vi "testserverstream.vi"() -> ()   [LabVIEW 2016]
uses:
  dllwrapper/tls data user event.ctl
  dllwrapper/tls new socket user event.ctl
  dllwrapper/tls action complete user event.ctl
  dllwrapper/async tls.lvlib
  lvasynctls.dll
panel:
  out "buffer":string
  out "streamreaderr":i32
  out "read size?":u64
  out "error string":string
  out "length":u32
  out "errstring":string
  out "anyconn 2":u32 format="%.0x"
  out "anyconn":u64 format="%.0x"
  out "options":errorcluster
  out "data":string
  out "bad connection":u64
  out "request type 3":u8 format="%.0x"
  out "request ID 3":u32 format="%.0x"
  out "error code 3":i32 format="%.0x"
  out "request type 2":u8 format="%.0x"
  out "request ID 2":u32 format="%.0x"
  out "error code 2":i32 format="%.0x"
  out "error code":i32
  out "request ID":u32 format="%.0x"
  out "request type":u32 format="%.0x"
  out "error out 10":errorcluster
  out "error out 9":errorcluster
  out "error out 6":errorcluster
  out "error out 5":errorcluster
  out "error out 4":errorcluster
  out "error out 3":errorcluster
  out "error out 2":errorcluster
  # "read result"
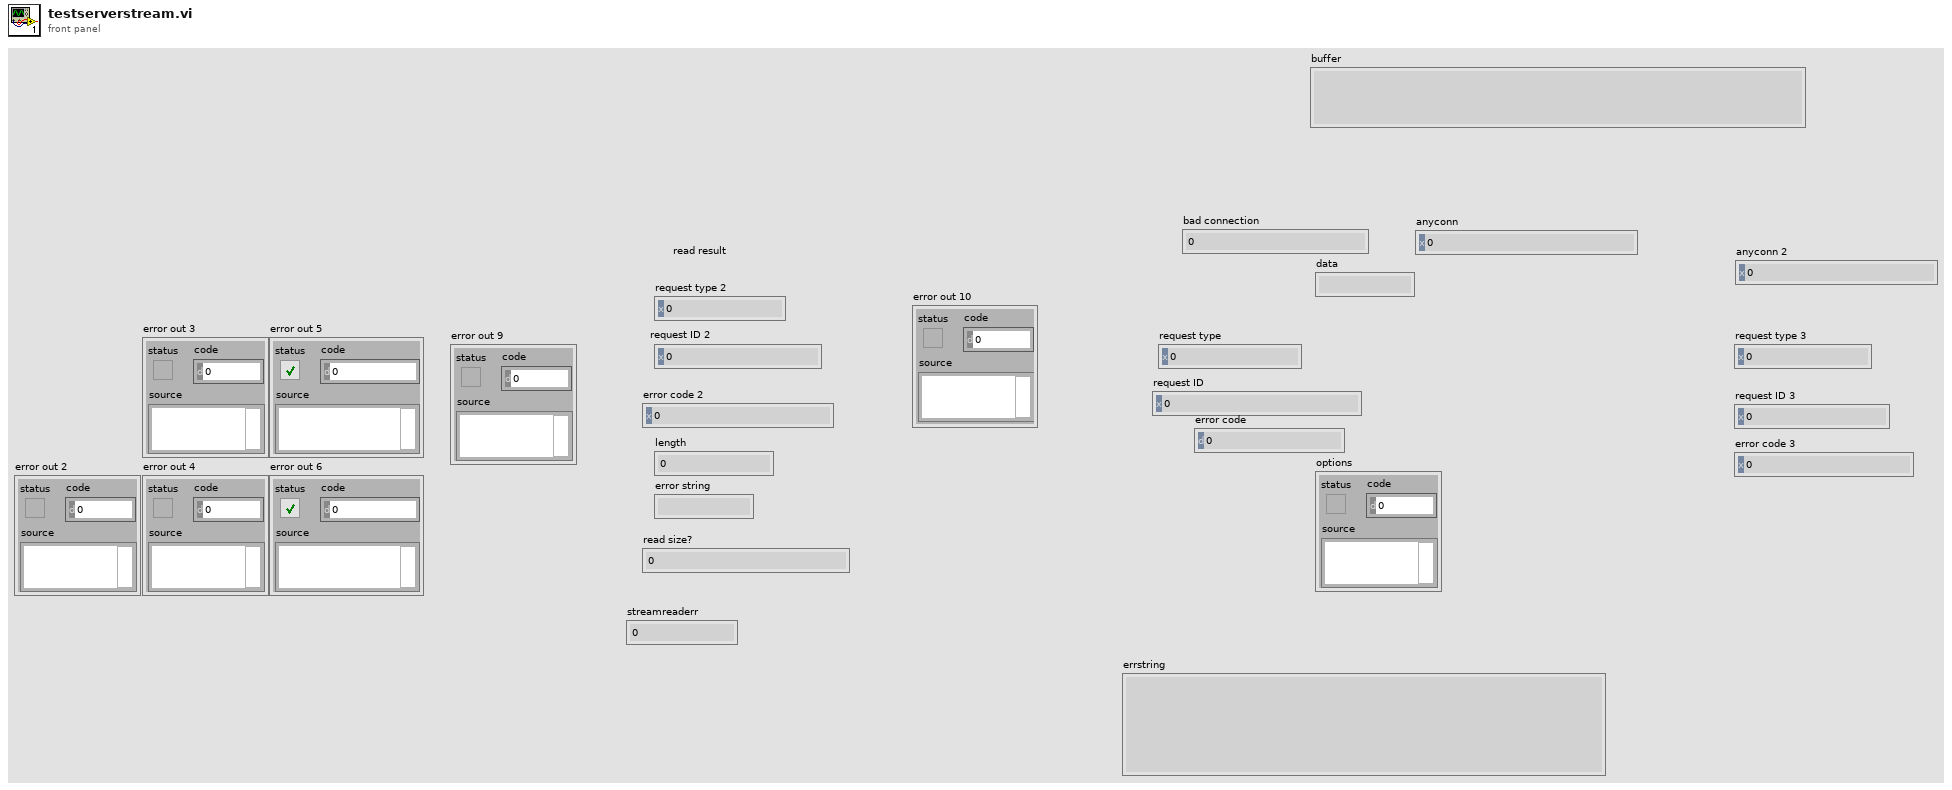
[diagram p1: front panel]
types:
  T1 = typedef "async tls.lvlib/tls action complete user event.ctl" = cluster{"request type":u8, "request ID":u32, "error code":i32, "error string":string, "length":u32}
  T2 = typedef "async tls.lvlib/tls new socket user event.ctl" = cluster{"request type":u32, "request ID":u32, "error code":i32, "errstring":string, "connection":u64}
  T3 = typedef "async tls.lvlib/tls data user event.ctl" = cluster{"request type":u8, "request ID":u32, "error code":i32, "data":string}
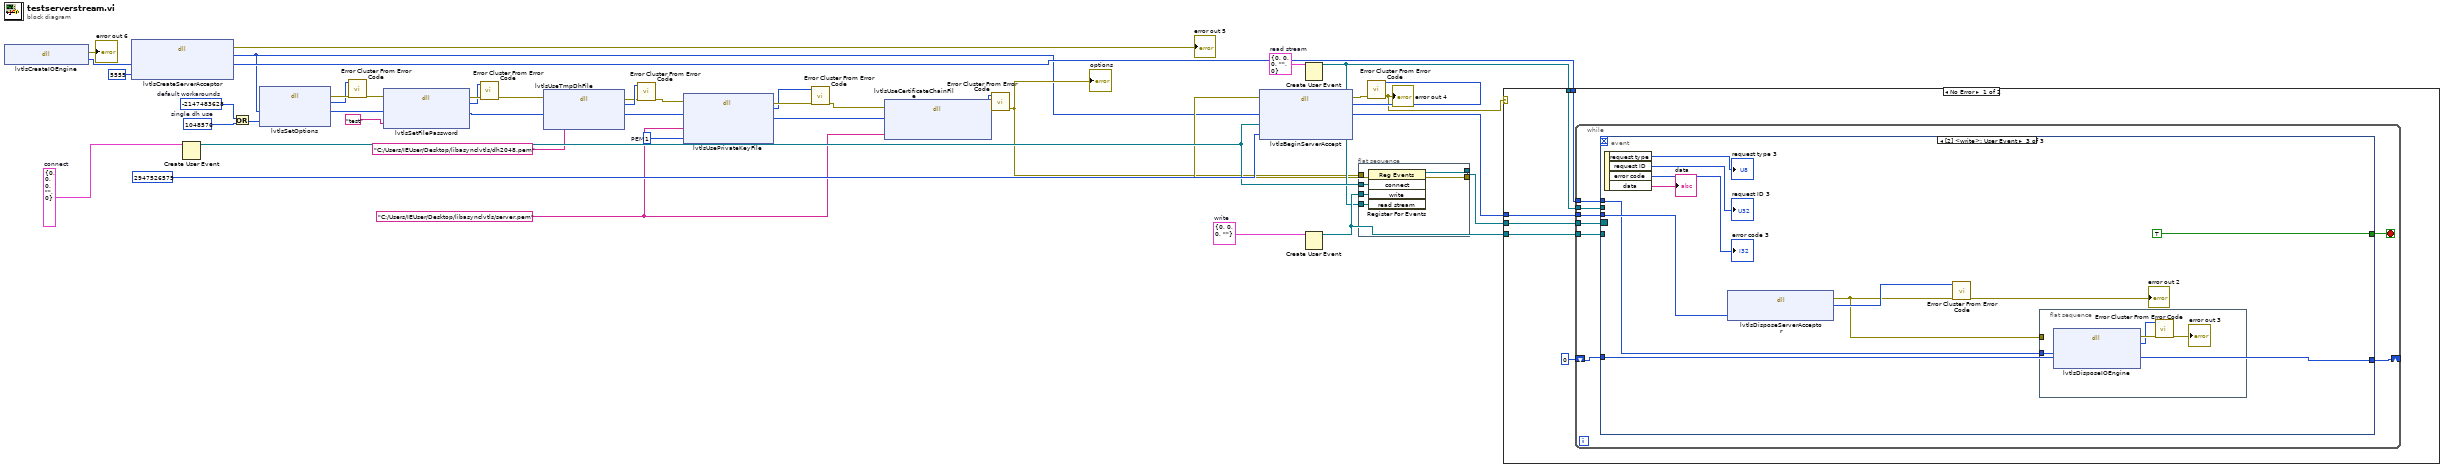
[diagram p0: block diagram]
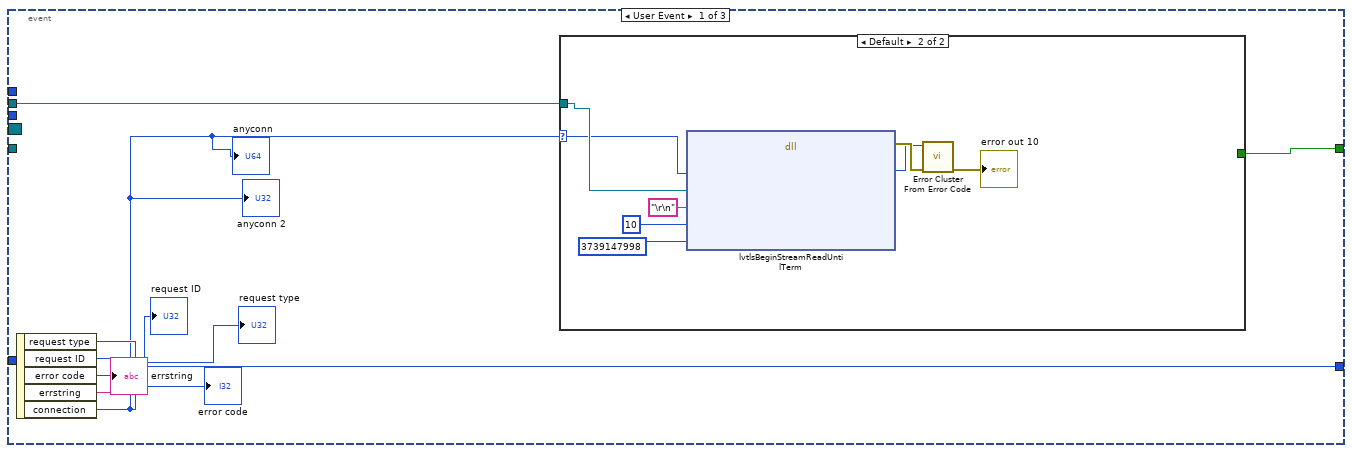
[diagram p2: hidden frame]
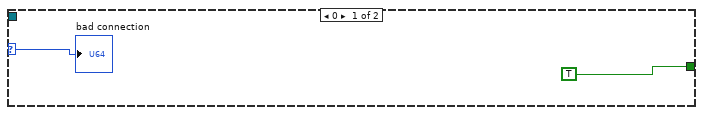
[diagram p3: hidden frame]
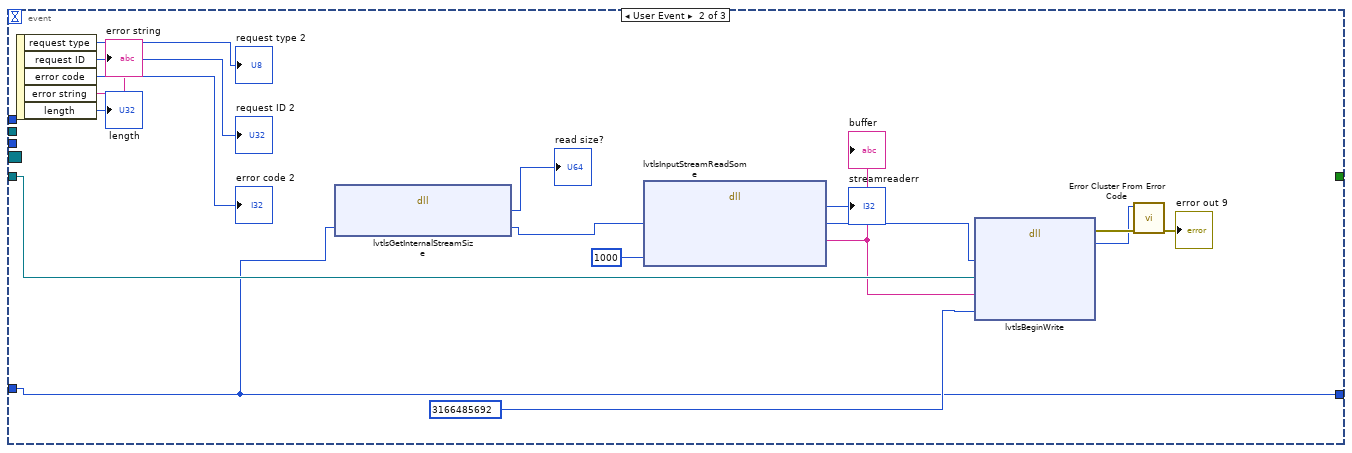
[diagram p4: hidden frame]
diagram:
  w1 = T1 {"request type"=0, "request ID"=0, "error code"=0, "error string"="", "length"=0}  # read stream
  w12 = "C:/Users/IEUser/Desktop/libasynclvtls/server.pem" ("file")
  w14 = 1  # PEM
  w15 = -2147483628  # default workarounds
  w16 = 1048576  # single dh use
  w33 = T2 {"request type"=0, "request ID"=0, "error code"=0, "errstring"="", "connection"=0}  # connect
  w39 = T3 {"request type"=0, "request ID"=0, "error code"=0, "data"=""}  # write
  n1 = dll-call lib="C:/Users/IEUser/Desktop/libasynclvtls/lvasynctls.dll" fn="lvtlsCreateIOEngine"() -> (error out=→"error out 6":errorcluster, "engine"=w45:u64)  [unwired: 3 in, 1 out]
  n2 = dll-call lib="C:/Users/IEUser/Desktop/libasynclvtls/lvasynctls.dll" fn="lvtlsCreateServerAcceptor"("engine"=w45, "port"=u16 5555) -> (error out=→"error out 5":errorcluster, "acceptor"=w3:u64, "engine"=w20:u64)  [unwired: 4 in, 1 out]
  n3 = Create User Event(user event datatype=w33) -> (user event=w36:refnum<user-event>)  [unwired: 1 in, 1 out]
  n4 = Or(x=w15, y=w16) -> (x .or. y?=w17:i32)
  n5 = dll-call lib="C:/Users/IEUser/Desktop/libasynclvtls/lvasynctls.dll" fn="lvtlsSetOptions"("connCreator"=w3, "options"=w17) -> (error out=w30:errorcluster, "err"=w29:i32, "connCreator"=w6:u64)  [unwired: 4 in, 1 out]
  n6 = call <vilib>:"Error Cluster From Error Code.vi"("error in (no error)"=w30, "error code (0)"=w29) -> ("error out"=w7:errorcluster)  [unwired: 7 in]
  n7 = dll-call lib="C:/Users/IEUser/Desktop/libasynclvtls/lvasynctls.dll" fn="lvtlsSetFilePassword"(error in=w7, "connCreator"=w6, "password"="test" ("file")) -> (error out=w10:errorcluster, "err"=w9:i32, "connCreator"=w5:u64)  [unwired: 3 in, 1 out]
  n8 = call <vilib>:"Error Cluster From Error Code.vi"("error in (no error)"=w10, "error code (0)"=w9) -> ("error out"=w8:errorcluster)  [unwired: 7 in]
  n9 = dll-call lib="C:/Users/IEUser/Desktop/libasynclvtls/lvasynctls.dll" fn="lvtlsUseTmpDhFile"(error in=w8, "connCreator"=w5, "file"="C:/Users/IEUser/Desktop/libasynclvtls/dh2048.pem") -> (error out=w27:errorcluster, "err"=w28:i32, "connCreator"=w19:u64)  [unwired: 3 in, 1 out]
  n10 = call <vilib>:"Error Cluster From Error Code.vi"("error in (no error)"=w27, "error code (0)"=w28) -> ("error out"=w21:errorcluster)  [unwired: 7 in]
  n11 = dll-call lib="C:/Users/IEUser/Desktop/libasynclvtls/lvasynctls.dll" fn="lvtlsUsePrivateKeyFile"(error in=w21, "connCreator"=w19, "file"=w12, "format"=w14) -> (error out=w26:errorcluster, "err"=w25:i32, "connCreator"=w18:u64)  [unwired: 4 in, 1 out]
  n12 = call <vilib>:"Error Cluster From Error Code.vi"("error in (no error)"=w26, "error code (0)"=w25) -> ("error out"=w22:errorcluster)  [unwired: 7 in]
  n13 = dll-call lib="C:/Users/IEUser/Desktop/libasynclvtls/lvasynctls.dll" fn="lvtlsUseCertificateChainFile"(error in=w22, "connCreator"=w18, "file"=w12) -> (error out=w23:errorcluster, "err"=w24:i32)  [unwired: 4 in, 1 out]
  n14 = call <vilib>:"Error Cluster From Error Code.vi"("error in (no error)"=w23, "error code (0)"=w24) -> ("error out"=w13:errorcluster)  [unwired: 7 in]
  "options" <- w13
  n15 = dll-call lib="C:/Users/IEUser/Desktop/libasynclvtls/lvasynctls.dll" fn="lvtlsBeginServerAccept"(error in=w32, "acceptor"=w3, "event"=w36, "id"=u32 2947526575 ("err")) -> (error out=w43:errorcluster, "err"=w38:i32, "acceptor"=w37:u64)  [unwired: 4 in, 1 out]
  n16 = Create User Event(user event datatype=w1) -> (user event=w34:refnum<user-event>)  [unwired: 1 in, 1 out]
  n17 = Create User Event(user event datatype=w39) -> (user event=w35:refnum<user-event>)  [unwired: 1 in, 1 out]
  n18 = flat-sequence {
    tunnel: [w50] -> w40
    tunnel: w36 -> [w49]
    tunnel: w35 -> [w48]
    tunnel: w34 -> [w47]
    tunnel: [w46] -> w32
    tunnel: w13 -> [_]
    frame #0 {
      n19 = register-events(w49, w48, w47) -> (reference out=w50:refnum<event-registration>, error out=w46:errorcluster)  [unwired: 2 in]
    }
  }
  n20 = call <vilib>:"Error Cluster From Error Code.vi"("error in (no error)"=w43, "error code (0)"=w38) -> ("error out"=w2:errorcluster)  [unwired: 7 in]
  "error out 4" <- w2
  n21 = case shown="No Error" w2 {
    tunnel: w40 -> [w56 _]
    tunnel: w37 -> [w55 _]
    tunnel: w35 -> [w54 _]
    tunnel: w34 -> [w53 _]
    tunnel: w20 -> [w51 _]
    frame No Error {
      n22 = while {
        tunnel: w56 -> [w64]
        tunnel: w54 -> [w62]
        tunnel: w55 -> [w61]
        tunnel: w53 -> [w60]
        tunnel: w51 -> [w59]
        shift-right: [w58] -> _
        shift-left: u32 0 -> [w57]
        stop <- w63 stop-if-true
        n23 = event shown="[2] <write>: User Event" {
          selector: w64 -> [_ _ _]
          dyn-events: _ -> [_ _ _]
          timeout: _ -> [_ _ _]
          tunnel: [w68 _ TRUE] -> w63
          tunnel: w62 -> [_ w91 _]
          tunnel: w61 -> [_ _ w103]
          tunnel: w60 -> [w67 _ _]
          tunnel: w59 -> [_ _ w102]
          tunnel: [w66 w88 w100] -> w58
          tunnel: w57 -> [_ w88 w100]
          event User Event {
            n24 = event-data() -> ("request type"=→"request type":u32, "request ID"=→"request ID":u32, "error code"=→"error code":i32, "errstring"=→"errstring":string, "connection"=w66:u64)  [unwired: 1 in]
            "anyconn" <- w66
            "anyconn 2" <- w66
            n25 = case shown="Default" w66 {
              selector: w66 -> [w72 w75]
              tunnel: [TRUE _] -> w68
              tunnel: w67 -> [_ w76]
              frame 0 {
                "bad connection" <- w72
              }
              frame Default {
                n26 = dll-call lib="C:/Users/IEUser/Desktop/libasynclvtls/lvasynctls.dll" fn="lvtlsBeginStreamReadUntilTerm"("socket"=w75, "event"=w76, "termination"="\r\n", "bytes to read"=10, "id"=u32 3739147998 ("err")) -> (error out=w80:errorcluster, "err"=w78:i32)  [unwired: 8 in, 1 out]
                n27 = call <vilib>:"Error Cluster From Error Code.vi"("error in (no error)"=w80, "error code (0)"=w78) -> ("error out"=→"error out 10":errorcluster)  [unwired: 7 in]
              }
            }
          }
          event User Event {
            n28 = event-data() -> ("request type"=→"request type 2":u8, "request ID"=→"request ID 2":u32, "error code"=→"error code 2":i32, "error string"=→"error string":string, "length"=→"length":u32)  [unwired: 1 in]
            n29 = dll-call lib="C:/Users/IEUser/Desktop/libasynclvtls/lvasynctls.dll" fn="lvtlsGetInternalStreamSize"("socket"=w88) -> ("size"=→"read size?":u64, "socket"=w86:u64)  [unwired: 3 in, 2 out]
            n30 = dll-call lib="C:/Users/IEUser/Desktop/libasynclvtls/lvasynctls.dll" fn="lvtlsInputStreamReadSome"("socket"=w86, "maxlen"=u64 1000) -> ("err"=→"streamreaderr":i32, "socket"=w85:u64, "buffer"=w82:string)  [unwired: 5 in, 2 out]
            "buffer" <- w82
            n31 = dll-call lib="C:/Users/IEUser/Desktop/libasynclvtls/lvasynctls.dll" fn="lvtlsBeginWrite"("socket"=w85, "event"=w91, "data"=w82, "requestID"=u32 3166485692 ("err")) -> (error out=w95:errorcluster, "err"=w93:i32)  [unwired: 7 in, 1 out]
            n32 = call <vilib>:"Error Cluster From Error Code.vi"("error in (no error)"=w95, "error code (0)"=w93) -> ("error out"=→"error out 9":errorcluster)  [unwired: 7 in]
          }
          event User Event {
            n33 = event-data() -> ("request type"=→"request type 3":u8, "request ID"=→"request ID 3":u32, "error code"=→"error code 3":i32, "data"=→"data":string)  [unwired: 1 in]
            n34 = dll-call lib="C:/Users/IEUser/Desktop/libasynclvtls/lvasynctls.dll" fn="lvtlsDisposeServerAcceptor"("acceptor"=w103) -> (error out=w101:errorcluster, "err"=w105:i32)  [unwired: 4 in, 1 out]
            n35 = call <vilib>:"Error Cluster From Error Code.vi"("error in (no error)"=w101, "error code (0)"=w105) -> ("error out"=→"error out 2":errorcluster)  [unwired: 7 in]
            n36 = flat-sequence {
              tunnel: w102 -> [w110]
              tunnel: w101 -> [_]
              frame #0 {
                n37 = dll-call lib="C:/Users/IEUser/Desktop/libasynclvtls/lvasynctls.dll" fn="lvtlsDisposeIOEngine"("engine"=w110) -> (error out=w113:errorcluster, "err"=w112:i32)  [unwired: 6 in, 1 out]
                n38 = call <vilib>:"Error Cluster From Error Code.vi"("error in (no error)"=w113, "error code (0)"=w112) -> ("error out"=→"error out 3":errorcluster)  [unwired: 7 in]
              }
            }
          }
        }
      }
    }
    frame Error {
    }
  }
